vi "Main.vi"() -> ()   [LabVIEW 2013]
uses:
  <vilib>/myRIO/Instrument Drivers/Onboard IO/UART/typedef/VISA Configuration.ctl
  <vilib>/myRIO/Common/Instrument Driver Framework/myRIO v1.0/UART/vis/myRIO v1.0 Close UART.vi
  <vilib>/Instr/_visa.llb/VISA Configure Serial Port (Instr).vi
  <vilib>/myRIO/Common/Instrument Driver Framework/Utilities/vis/FPGA Ref Manager.vi
  <vilib>/myRIO/Common/Instrument Driver Framework/myRIO v1.0/myRIO v1.0 Reset FPGA.vi
  <vilib>/myRIO/Instrument Drivers/Utilities/Utilities.lvlib
  <vilib>/myRIO/Instrument Drivers/Onboard IO/UART/UART.lvlib
panel:
  in  "error in (no error)":errorcluster
  in  "stop (F)":bool caption="Stop"
  out "Heart Rate [bpm] 2":u32
  out "Heart Rate [bpm]":dbl(knob) scale=0.0..220.0
  out "error out":errorcluster
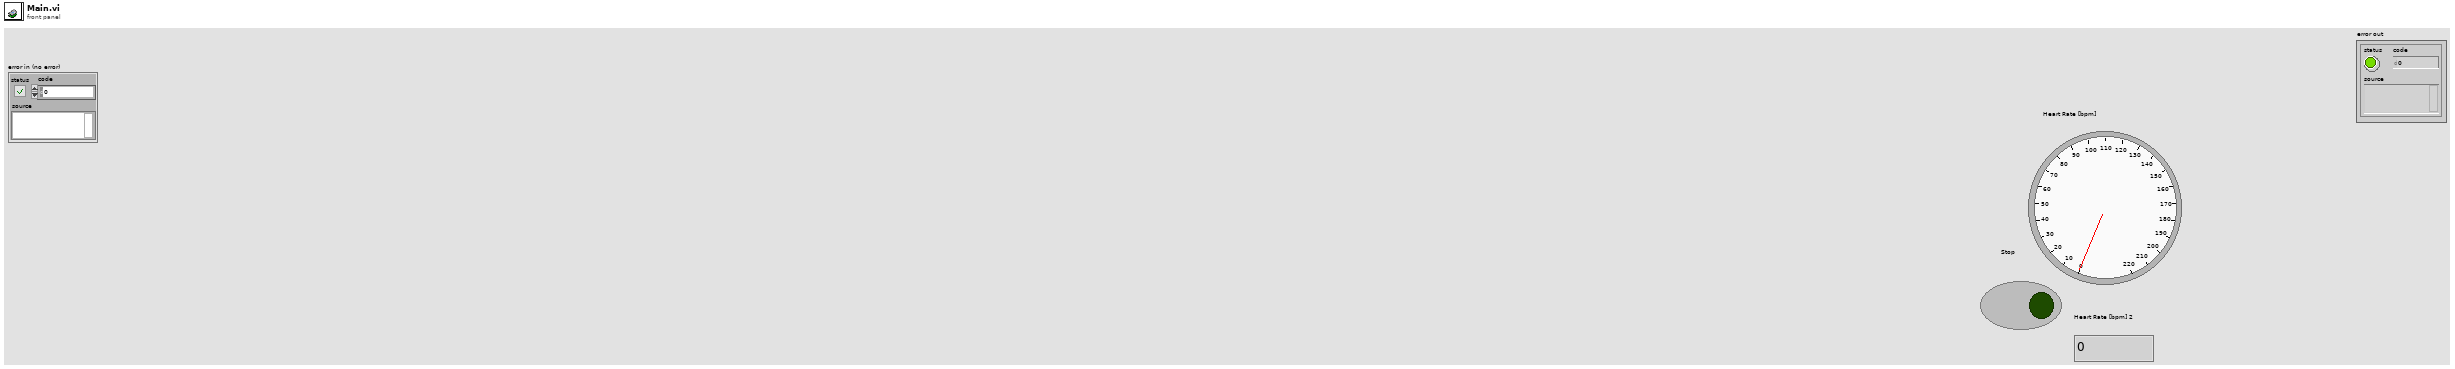
[diagram p1: front panel]
types:
  T1 = typedef "UART.lvlib/VISA Configuration.ctl" = cluster{"baud rate (9600)":u32, "data bits (8)":u16, "parity (0:none)":enum16{"None", "Odd", "Even", "Mark", "Space"}, "stop bits (10: 1 bit)":u16, "flow control (0:none)":u16, "termination char\n(0xA = '\\n' = LF) ":u8, "Enable Termination\nChar (T)":bool, "timeout (10sec)":u32}
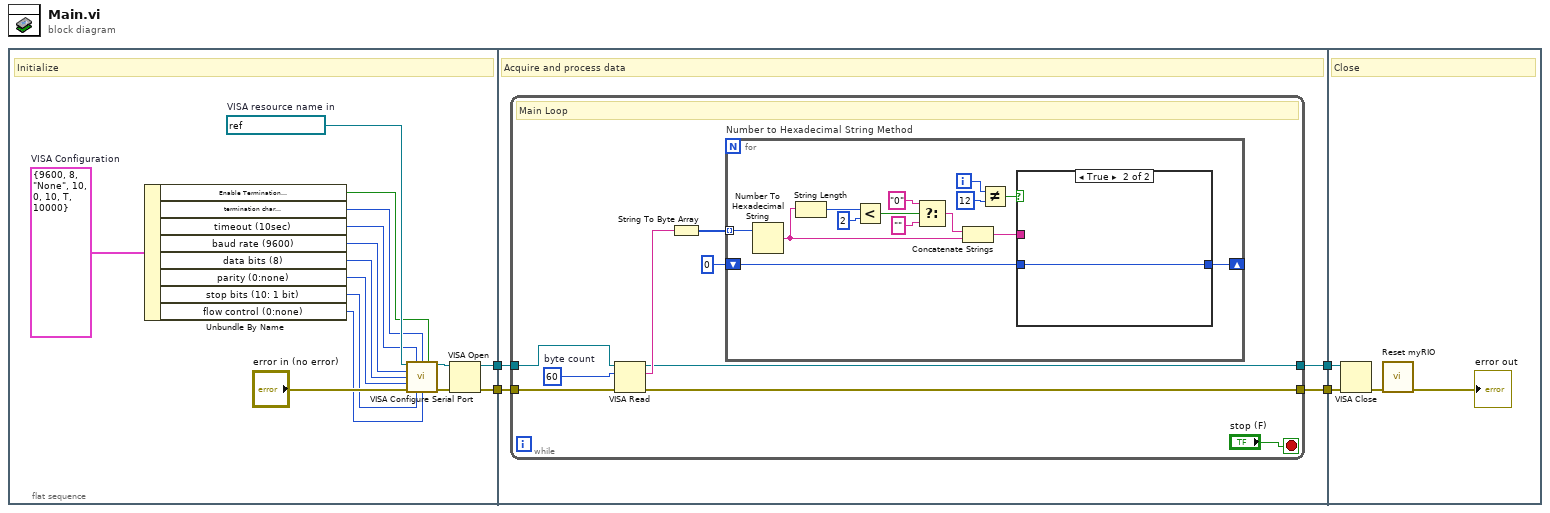
[diagram p0: block diagram]
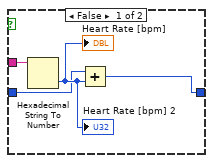
[diagram p2: hidden frame]
diagram:
  n1 = flat-sequence {
    tunnel: [w19] -> w3
    tunnel: [w18] -> w2
    tunnel: [w23] -> w4
    tunnel: w3 -> [w21]
    tunnel: w2 -> [w20]
    tunnel: [w22] -> w1
    tunnel: w4 -> [w53]
    tunnel: w1 -> [w52]
    frame #0 {
      w16 = T1 {"baud rate (9600)"=9600, "data bits (8)"=8, "parity (0:none)"=enum."None", "stop bits (10: 1 bit)"=10, "flow control (0:none)"=0, "termination char\n(0xA = '\\n' = LF) "=10, "Enable Termination\nChar (T)"=TRUE, "timeout (10sec)"=10000}  # VISA Configuration
      w17 = refnum<visa-resource-name> "ASRL1::INSTR"  # VISA resource name in
      # "Initialize"
      n2 = Unbundle By Name(w16) -> ("Enable Termination\nChar (T)"=w14:bool, "termination char\n(0xA = '\\n' = LF)"=w13:u8, "timeout (10sec)"=w12:u32, "baud rate (9600)"=w7:u32, "data bits (8)"=w8:u16, "parity (0:none)"=w9:enum16{"None", "Odd", "Even", "Mark", "Space"}, "stop bits (10: 1 bit)"=w10:u16, "flow control (0:none)"=w11:u16)
      n3 = call-poly "VISA Configure Serial Port"("VISA resource name"=w17, "timeout (10sec)"=w12, "termination char\n(0xA = '\\n' = LF)"=w13, "Enable Termination\nChar (T)"=w14, "baud rate (9600)"=w7, "data bits (8)"=w8, "parity (0:none)"=w9, "error in (no error)"="error in (no error)", "stop bits (10: 1 bit)"=w10, "flow control (0:none)"=w11) -> ("VISA resource name out"=w6:refnum<visa-resource-name>, "error out"=w5:errorcluster)  [unwired: 4 in]
      n4 = VISA Open(error in (no error)=w5, VISA resource name=w6) -> (VISA resource name=w19:refnum<visa-resource-name>, error out=w18:errorcluster)  [unwired: 3 in]
    }
    frame #1 {
      # "Acquire and process data"
      n5 = while {
        tunnel: w20 -> [w27]
        tunnel: w21 -> [w28]
        tunnel: [w25] -> w23
        tunnel: [w24] -> w22
        stop <- "stop (F)" stop-if-true
        w29 = u32 60  # byte count
        # "Main Loop"
        n6 = VISA Read(VISA resource name=w28, byte count=w29, error in (no error)=w27) -> (VISA resource name out=w25:refnum<visa-resource-name>, read buffer=w26:string, error out=w24:errorcluster)  [unwired: 1 out]
        n7 = String To Byte Array(string=w26) -> (unsigned byte array=w32:u8[])
        n8 = for "Number to Hexadecimal String Method" {
          tunnel: w32 -> [w42] mode=indexing
          shift-right: [w35] -> _
          shift-left: u32 0 -> [w34]
          i -> [w39]
          n9 = Number To Hexadecimal String(2:w42) -> (0:w33:string)  [unwired: 1 in]
          n10 = String Length(string=w33) -> (length=w46:i32)
          n11 = Less?(x=w46, y=2) -> (x < y?=w44:bool)
          n12 = Select(t="0", s=w44, f="") -> (s? t:f=w40:string)
          n13 = Concatenate Strings(w40, w33) -> (w36:string)
          n14 = Not Equal?(x=w39, y=12) -> (x != y?=w37:bool)
          n15 = case shown="True" w37 {
            tunnel: w36 -> [w50 _]
            tunnel: [w48 w51] -> w35
            tunnel: w34 -> [w47 w51]
            frame False {
              n16 = Hexadecimal String To Number(string=w50) -> (number=w49:u32)  [unwired: 2 in, 1 out]
              "Heart Rate [bpm] 2" <- w49
              "Heart Rate [bpm]" <- w49
              n17 = Add(x=w47, y=w49) -> (x+y=w48:u32)
            }
            frame True {
            }
          }
        }
      }
    }
    frame #2 {
      # "Close"
      n18 = VISA Close(VISA resource name=w53, error in (no error)=w52) -> (error out=w54:errorcluster)
      n19 = call <vilib>:"Reset myRIO.vi"("error in (no error)"=w54) -> ("error out"=→"error out":errorcluster)  [unwired: 10 in]
    }
  }
